vi "SCAN from String.vi"() -> ()   [LabVIEW 2022 SP3]
panel:
  out "output 4":string
  out "output 3":i32
  out "output 2":string
  out "output 1":string
  in  "String":string
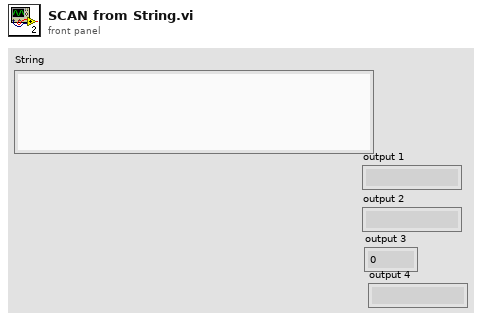
[diagram p1: front panel]
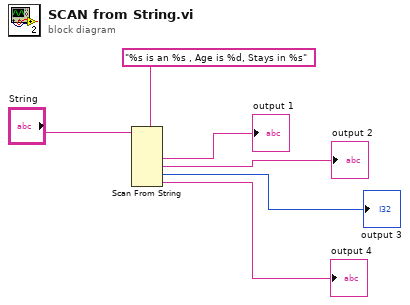
[diagram p0: block diagram]
diagram:
  n1 = Scan From String(format string="%s is an %s , Age is %d, Stays in %s", input string="String") -> (output 1=→"output 1":string, output 2=→"output 2":string, output 3=→"output 3":i32, output 4=→"output 4":string)  [unwired: 6 in, 3 out]
